vi "Main On Compile Action VI_Parse BC.vi"(7 "Autocreate Rx timestamp chans?":bool, 8 "error in":errorcluster, 10 "Channel Ref":u64, 11 "Device Item Ref in":T2 format="%.0x") -> (0 "error out":errorcluster, 2 "Channel Ref":u64, 3 "BC":T1 {"Acyclic Frames Trigger Channels Refs" format="%.0x"; "Command Channels Refs" format="%.0x"; "messages"."Timestamp Channel Data Reference" format="%.0x"; "messages"."Status Channel Data Refs" format="%.0x"; "messages"."Words Item Refs" format="%.0x"; "messages"."Words Block Data Refs"."Data Reference" format="%.0x"})   [LabVIEW 2017, in "Ballard 1553 System Explorer.lvlib"]
uses:
  Ballard 1553 System Explorer.lvlib
  <vilib>/NI Veristand/Custom Device API/Custom Device Item Ref.ctl
  Shared/Controls and Global/RT BC.ctl
  Shared/Controls and Global/RT Message.ctl
  Shared/Controls and Global/RT messageType.ctl
  Shared/Controls and Global/RT CWD1.ctl
  Shared/Controls and Global/RT CWD2.ctl
  <vilib>/NI Veristand/Custom Device API/Data Reference.ctl
  <vilib>/NI Veristand/Custom Device API/Block Data Reference.ctl
  Parse XML Ballard/Ballard_messageType.ctl
  Parse XML Ballard/Ballard_CWD1.ctl
  Parse XML Ballard/Ballard_CWD2.ctl
  <vilib>/NI Veristand/Custom Device API/Data Access Type.ctl
  Shared/Controls and Global/Global.vi
  <vilib>/NI Veristand/Custom Device Tools/Custom Device Utility Library/NI VeriStand - Search for Item by GUID.vi
  <vilib>/NI Veristand/Custom Device API/Get Item Property (I32).vi
  <vilib>/NI Veristand/Custom Device API/Get Item Property (String).vi
  <vilib>/NI Veristand/Custom Device Tools/Custom Device Utility Library/NI VeriStand - Search for Item by Name.vi
  <vilib>/NI Veristand/Custom Device Tools/Custom Device Utility Library/NI VeriStand - Search for All Items by GUID.vi
  <vilib>/NI Veristand/Custom Device API/Get Item Property (U16).vi
  <vilib>/NI Veristand/Custom Device API/Get Item Property (Variant).vi
  Shared/Ballard 1553 Shared.lvlib
  <vilib>/NI VeriStand/Custom Device Tools/Custom Device Utility Library/Custom Device Utility Library.lvlib
  <vilib>/NI VeriStand/Custom Device API/Custom Device API.lvlib
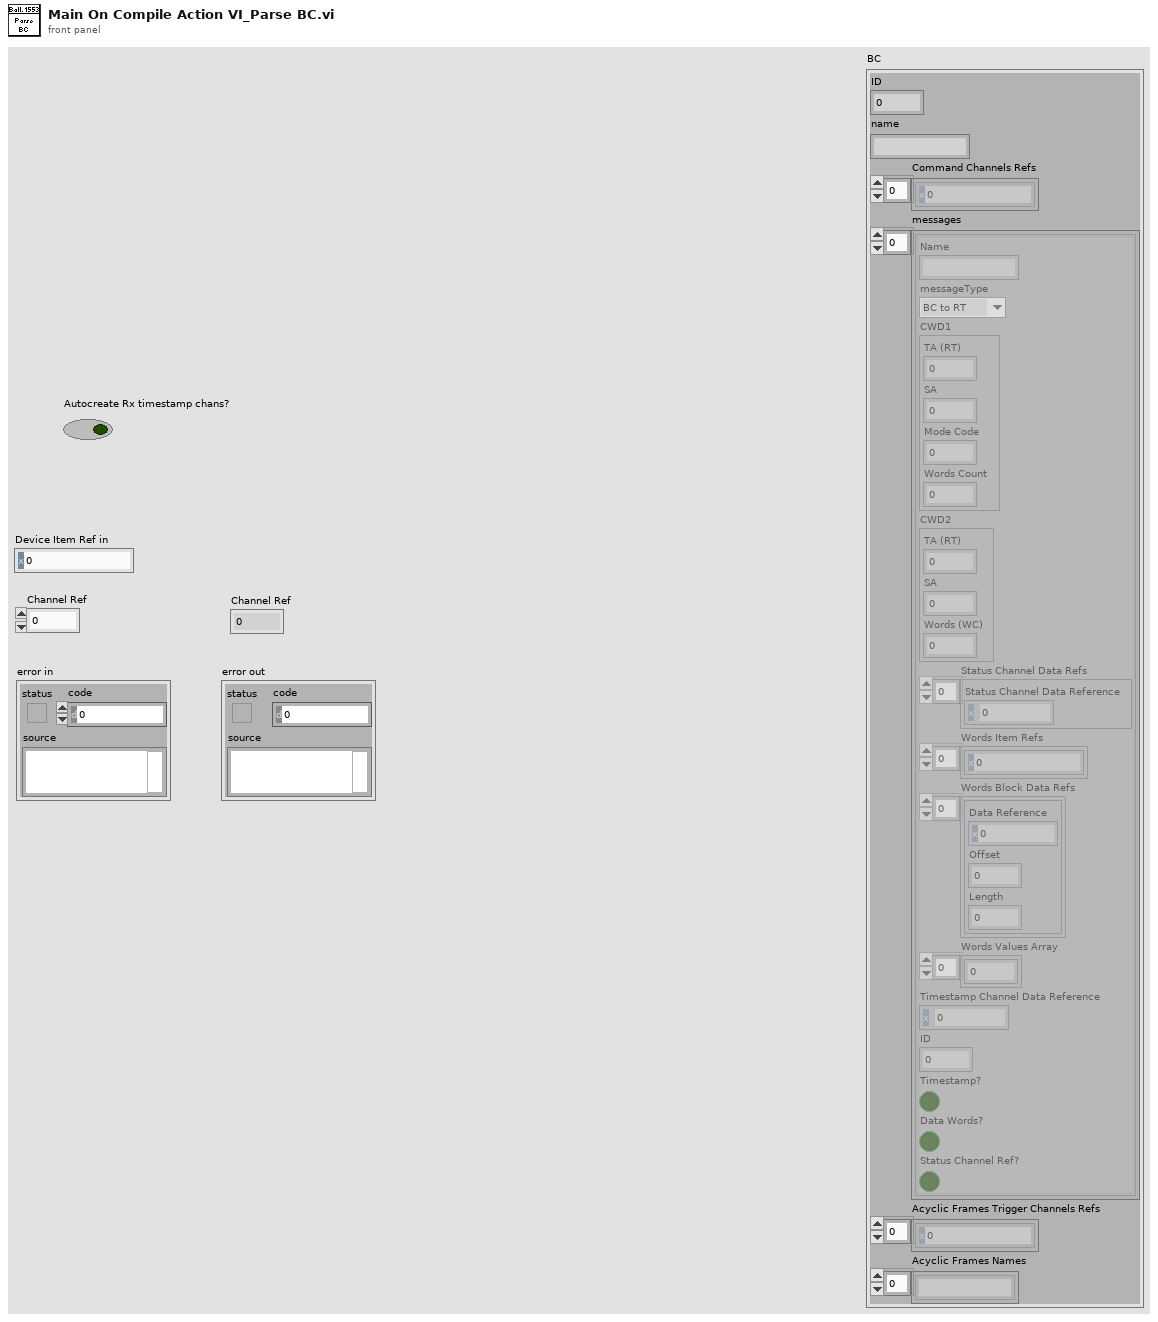
[diagram p1: front panel]
types:
  T1 = typedef "Ballard 1553 Shared.lvlib/RT BC.ctl" = cluster{"ID":i32, "name":string, "Command Channels Refs":T2[], "messages":T3[], "Acyclic Frames Trigger Channels Refs":T2[], "Acyclic Frames Names":string[]}
  T2 = typedef "Custom Device API.lvlib/Custom Device Item Ref.ctl" = u64
  T3 = typedef "Ballard 1553 Shared.lvlib/RT Message.ctl" = cluster{"Name":string, "messageType":T4, "CWD1":T5, "CWD2":T6, "Status Channel Data Refs":T7[], "Words Item Refs":T2[], "Words Block Data Refs":T8[], "Words Values Array":u16[], "Timestamp Channel Data Reference":T7, "ID":i32, "Timestamp?":bool, "Data Words?":bool, "Status Channel Ref?":bool}
  T4 = typedef "Ballard 1553 Shared.lvlib/RT messageType.ctl" = enum16{"BC to RT", "RT to BC", "RT to RT", "MC (Rx)", "MC (Tx)"}
  T5 = typedef "Ballard 1553 Shared.lvlib/RT CWD1.ctl" = cluster{"TA (RT)":i8, "SA":i8, "Mode Code":i8, "Words Count":i8}
  T6 = typedef "Ballard 1553 Shared.lvlib/RT CWD2.ctl" = cluster{"TA (RT)":i8, "SA":i8, "Words (WC)":i8}
  T7 = typedef "Custom Device API.lvlib/Data Reference.ctl" = i32
  T8 = typedef "Custom Device API.lvlib/Block Data Reference.ctl" = cluster{"Data Reference":T7, "Offset":u64, "Length":u64}
  T9 = typedef "Ballard 1553 System Explorer.lvlib/Ballard_CWD2.ctl" = cluster{"TA (RT)":i8, "SA":i8, "Words (WC)":i8}
  T10 = typedef "Ballard 1553 System Explorer.lvlib/Ballard_CWD1.ctl" = cluster{"TA (RT)":i8, "SA":i8, "Mode Code":i8, "Words Count":i8}
  T11 = typedef "Ballard 1553 System Explorer.lvlib/Ballard_messageType.ctl" = enum16{"BC to RT", "RT to BC", "RT to RT", "MC (Rx)", "MC (Tx)"}
  T12 = typedef "Custom Device API.lvlib/Data Access Type.ctl" = enum16{"Read", "Write"}
  T13 = typedef "Custom Device API.lvlib/Custom Device Item Info.ctl" = cluster{"Name":string, "Is Channel":bool, "GUID":string, "Is Waveform":bool}
  T14 = typedef "Custom Device API.lvlib/Custom Device Channel.ctl" = cluster{"Type":T15, "Units":string, "Default Value":dbl, "Faultable":bool, "Scalable":bool}
  T15 = typedef "Custom Device API.lvlib/Custom Device Channel Type.ctl" = enum16{"Input", "Output"}
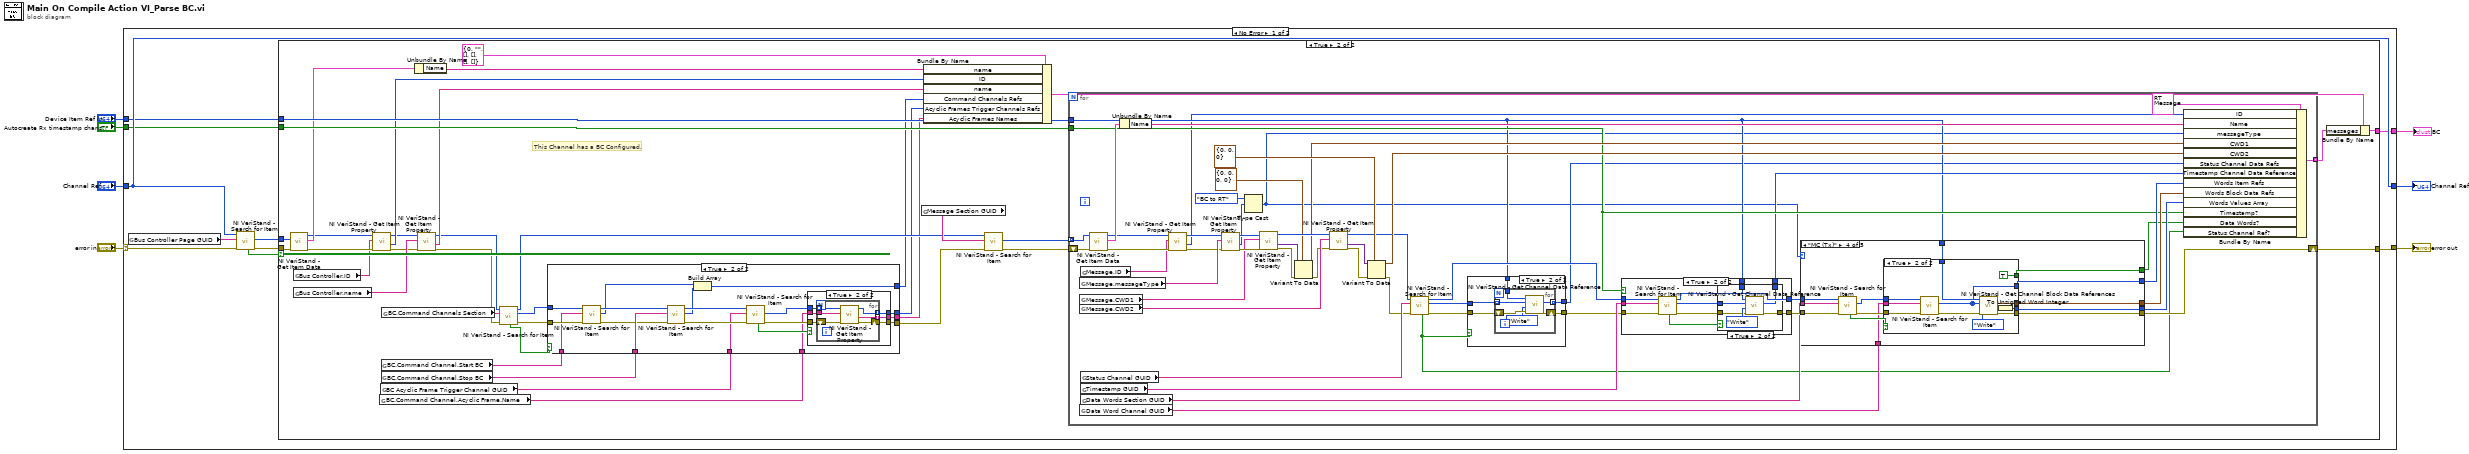
[diagram p0: block diagram]
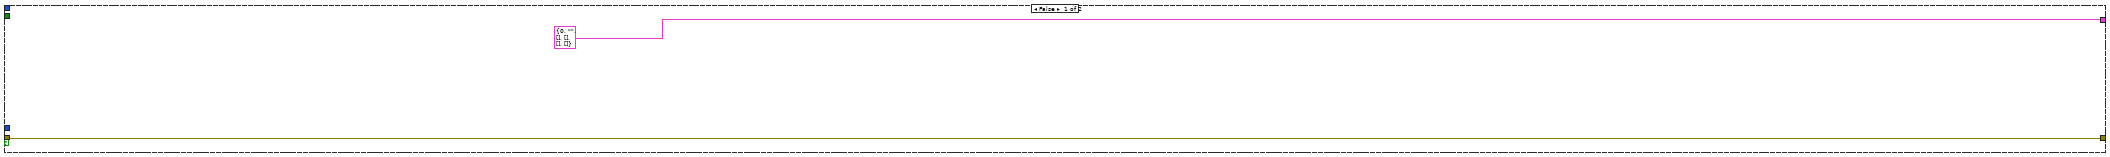
[diagram p2: hidden frame]
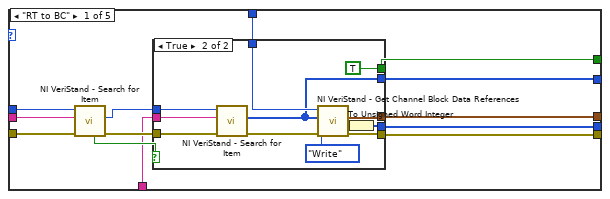
[diagram p6: hidden frame]
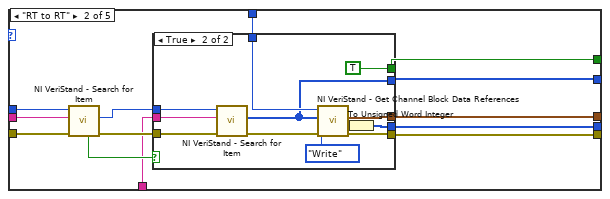
[diagram p8: hidden frame]
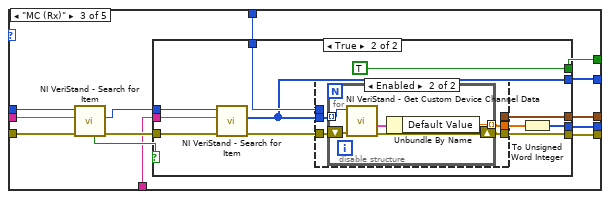
[diagram p10: hidden frame]
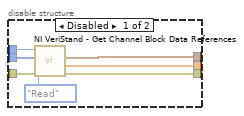
[diagram p12: hidden frame]
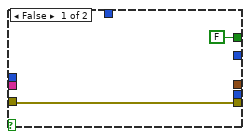
[diagram p13: hidden frame]
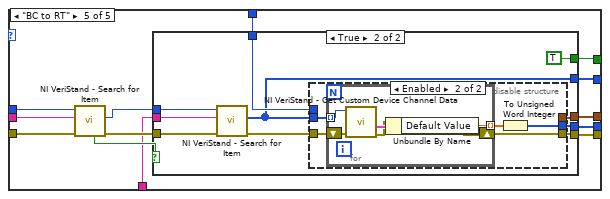
[diagram p14: hidden frame]
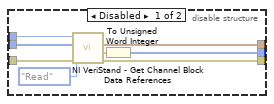
[diagram p16: hidden frame]
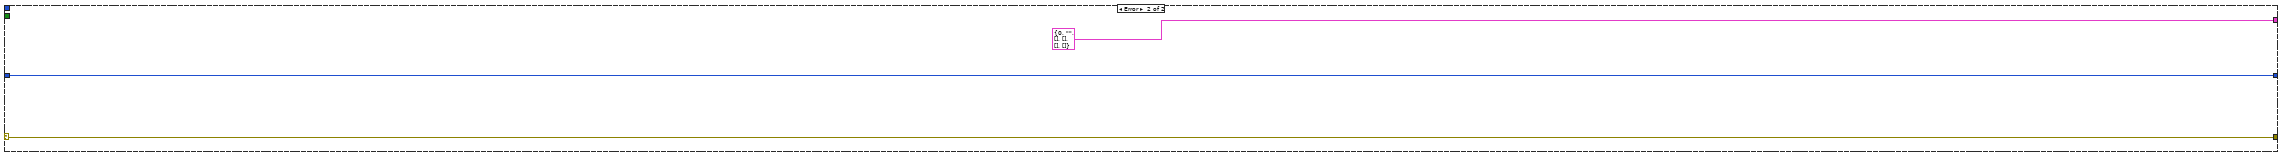
[diagram p19: hidden frame]
diagram:
  n1 = case shown="No Error" "error in" {
    selector: "error in" -> [w16 w338]
    tunnel: [w17 w338] -> w6
    tunnel: "Channel Ref" -> [w14 w337]
    tunnel: [w14 w337] -> w4
    tunnel: "Autocreate Rx timestamp chans?" -> [w10 _]
    tunnel: "Device Item Ref in" -> [w9 _]
    tunnel: [w8 T1 {"ID"=0, "name"="", "Command Channels Refs"=[], "messages"=[], "Acyclic Frames Trigger Channels Refs"=[], "Acyclic Frames Names"=[]} ("BC")] -> w1
    frame No Error {
      n2 = global read "Global.vi" "Bus Controller Page GUID"() -> (w15:string)
      n3 = call-poly <vilib>:"NI VeriStand - Search for Item.vi"("error in"=w16, "Item GUID"=w15, "Section Ref in"=w14) -> ("error out"=w13:errorcluster, "Item Ref"=w11:T2, "Found"=w12:bool)  [unwired: 5 in, 1 out]
      n4 = case shown="True" w12 {
        tunnel: w13 -> [w19 w39]
        tunnel: w11 -> [_ w40]
        tunnel: w10 -> [_ w53]
        tunnel: [w19 w52] -> w17
        tunnel: w9 -> [_ w51]
        tunnel: [T1 {"ID"=0, "name"="", "Command Channels Refs"=[], "messages"=[], "Acyclic Frames Trigger Channels Refs"=[], "Acyclic Frames Names"=[]} ("BC") w49] -> w8
        frame False {
        }
        frame True {
          # "This Channel has a BC Configured."
          n5 = call <vilib>:"NI VeriStand - Get Item Data.vi"("error in (no error)"=w39, "Item Ref in"=w40) -> ("error out"=w33:errorcluster, "Item Info"=w38:T13, "Item Ref out"=w34:T2)  [unwired: 6 in, 1 out]
          n6 = global read "Global.vi" "Bus Controller.ID"() -> (w32:string)
          n7 = global read "Global.vi" "Bus Controller.name"() -> (w29:string)
          n8 = call-poly <vilib>:"NI VeriStand - Get Item Property.vi"("error in (no error)"=w33, "Property Name"=w32, "Item Ref in"=w34) -> ("error out"=w28:errorcluster, "Value"=w31:i32, "Item Ref out"=w30:T2)  [unwired: 5 in, 1 out]
          n9 = global read "Global.vi" "BC.Command Channel.Acyclic Frame.Name"() -> (w22:string)
          n10 = global read "Global.vi" "BC Acyclic Frame Trigger Channel GUID"() -> (w23:string)
          n11 = global read "Global.vi" "BC.Command Channel.Start BC"() -> (w43:string)
          n12 = global read "Global.vi" "BC.Command Channel.Stop BC"() -> (w42:string)
          n13 = global read "Global.vi" "BC.Command Channels Section"() -> (w45:string)
          n14 = Unbundle By Name(w38) -> ("Name"=w36:string)
          n15 = call-poly <vilib>:"NI VeriStand - Get Item Property.vi"("error in (no error)"=w28, "Property Name"=w29, "Item Ref in"=w30) -> ("error out"=w27:errorcluster, "Value"=w26:string, "Item Ref out"=w24:T2)  [unwired: 5 in, 1 out]
          n16 = call-poly <vilib>:"NI VeriStand - Search for Item.vi"("error in"=w27, "Item Name"=w45, "Section Ref in"=w24) -> ("error out"=w46:errorcluster, "Item Ref"=w48:T2, "Section Ref out"=w41:T2, "Found"=w47:bool)  [unwired: 5 in]
          n17 = case shown="True" w47 {
            tunnel: w46 -> [w57 w76]
            tunnel: w48 -> [_ w75]
            tunnel: w43 -> [_ w74]
            tunnel: w42 -> [_ w73]
            tunnel: [w57 w61] -> w44
            tunnel: [_ w70] -> w25
            tunnel: [_ w60] -> w21
            tunnel: w23 -> [_ w68]
            tunnel: [_ w59] -> w20
            tunnel: w22 -> [_ w58]
            frame False {
            }
            frame True {
              n18 = call-poly <vilib>:"NI VeriStand - Search for Item.vi"("error in"=w76, "Item Name"=w74, "Section Ref in"=w75) -> ("error out"=w71:errorcluster, "Item Ref"=w66:T2, "Section Ref out"=w72:T2)  [unwired: 5 in, 1 out]
              n19 = call-poly <vilib>:"NI VeriStand - Search for Item.vi"("error in"=w71, "Item Name"=w73, "Section Ref in"=w72) -> ("error out"=w69:errorcluster, "Item Ref"=w65:T2, "Section Ref out"=w67:T2)  [unwired: 5 in, 1 out]
              n20 = Build Array(w66, w65) -> (w70:T2[])
              n21 = call-poly <vilib>:"NI VeriStand - Search for Item.vi"("error in"=w69, "Item GUID"=w68, "Section Ref in"=w67) -> ("error out"=w63:errorcluster, "Item Refs"=w62:T2[], "Found"=w64:bool)  [unwired: 5 in, 1 out]
              n22 = case shown="True" w64 {
                tunnel: w63 -> [w78 w83]
                tunnel: w62 -> [w77 w84]
                tunnel: [w78 w82] -> w61
                tunnel: [w77 w81] -> w60
                tunnel: [_ w80] -> w59
                tunnel: w58 -> [_ w79]
                frame False {
                }
                frame True {
                  n23 = for {
                    tunnel: w84 -> [w90] mode=indexing
                    shift-right: [w88] -> w82
                    shift-left: w83 -> [w89]
                    tunnel: [w87] -> w81 mode=indexing
                    tunnel: [w86] -> w80 mode=indexing
                    tunnel: w79 -> [w85]
                    n24 = call-poly <vilib>:"NI VeriStand - Get Item Property.vi"("error in (no error)"=w89, "Property Name"=w85, "Item Ref in"=w90) -> ("error out"=w88:errorcluster, "Value"=w86:string, "Item Ref out"=w87:T2)  [unwired: 5 in, 1 out]
                  }
                }
              }
            }
          }
          n25 = global read "Global.vi" "Message Section GUID"() -> (w56:string)
          n26 = Bundle By Name(cluster=T1 {"ID"=0, "name"="", "Command Channels Refs"=[], "messages"=[], "Acyclic Frames Trigger Channels Refs"=[], "Acyclic Frames Names"=[]} ("BC"), "name"=w36, "ID"=w31, "name"=w26, "Command Channels Refs"=w25, "Acyclic Frames Trigger Channels Refs"=w21, "Acyclic Frames Names"=w20) -> (w35:T1)
          n27 = call-poly <vilib>:"NI VeriStand - Search for Item.vi"("error in"=w44, "Item GUID"=w56, "Section Ref in"=w41) -> ("error out"=w55:errorcluster, "Item Refs"=w54:T2[])  [unwired: 5 in, 2 out]
          n28 = for {
            tunnel: w54 -> [w119] mode=indexing
            shift-right: [w121] -> w52
            shift-left: w55 -> [w120]
            tunnel: w53 -> [w102]
            tunnel: w51 -> [w94]
            tunnel: [w111] -> w50 mode=indexing
            n29 = global read "Global.vi" "Message.messageType"() -> (w139:string)
            n30 = global read "Global.vi" "Message.CWD1"() -> (w138:string)
            n31 = global read "Global.vi" "Message.CWD2"() -> (w137:string)
            n32 = global read "Global.vi" "Data Word Channel GUID"() -> (w122:string)
            n33 = global read "Global.vi" "Message.ID"() -> (w105:string)
            n34 = global read "Global.vi" "Status Channel GUID"() -> (w127:string)
            n35 = global read "Global.vi" "Timestamp GUID"() -> (w126:string)
            n36 = global read "Global.vi" "Data Words Section GUID"() -> (w123:string)
            n37 = call <vilib>:"NI VeriStand - Get Item Data.vi"("error in (no error)"=w120, "Item Ref in"=w119) -> ("error out"=w106:errorcluster, "Item Info"=w118:T13, "Item Ref out"=w107:T2)  [unwired: 6 in, 1 out]
            n38 = Unbundle By Name(w118) -> ("Name"=w117:string)
            n39 = call-poly <vilib>:"NI VeriStand - Get Item Property.vi"("error in (no error)"=w106, "Property Name"=w105, "Item Ref in"=w107) -> ("error out"=w104:errorcluster, "Value"=w91:i32, "Item Ref out"=w103:T2)  [unwired: 5 in, 1 out]
            n40 = call-poly <vilib>:"NI VeriStand - Get Item Property.vi"("error in (no error)"=w104, "Property Name"=w139, "Item Ref in"=w103) -> ("error out"=w142:errorcluster, "Value"=w131:u16, "Item Ref out"=w140:T2)  [unwired: 5 in, 1 out]
            n41 = Type Cast(type=Ballard_messageType."BC to RT" ("messageType"), x=w131) -> (*(type *) &x=w92:T11)
            n42 = call-poly <vilib>:"NI VeriStand - Get Item Property.vi"("error in (no error)"=w142, "Property Name"=w138, "Item Ref in"=w140) -> ("error out"=w136:errorcluster, "Value"=w133:variant, "Item Ref out"=w141:T2)  [unwired: 5 in, 1 out]
            n43 = Variant To Data(error in=w136, type=T10 {"TA (RT)"=0, "SA"=0, "Mode Code"=0, "Words Count"=0} ("CWD1"), Variant=w133) -> (data=w116:T10, error out=w134:errorcluster)
            n44 = call-poly <vilib>:"NI VeriStand - Get Item Property.vi"("error in (no error)"=w134, "Property Name"=w137, "Item Ref in"=w141) -> ("error out"=w135:errorcluster, "Value"=w132:variant, "Item Ref out"=w110:T2)  [unwired: 5 in, 1 out]
            n45 = Variant To Data(error in=w135, type=T9 {"TA (RT)"=0, "SA"=0, "Words (WC)"=0} ("CWD1"), Variant=w132) -> (data=w115:T9, error out=w109:errorcluster)
            n46 = call-poly <vilib>:"NI VeriStand - Search for Item.vi"("error in"=w109, "Item GUID"=w127, "Section Ref in"=w110) -> ("error out"=w98:errorcluster, "Item Refs"=w96:T2[], "Section Ref out"=w95:T2, "Found"=w99:bool)  [unwired: 5 in]
            n47 = case shown="True" w99 {
              tunnel: w98 -> [w143 w148]
              tunnel: [w143 w147] -> w97
              tunnel: w96 -> [_ w145]
              tunnel: w94 -> [_ w146]
              tunnel: [_ w144] -> w93
              frame False {
              }
              frame True {
                n48 = for {
                  tunnel: w146 -> [w152]
                  shift-right: [w153] -> w147
                  shift-left: w148 -> [w154]
                  tunnel: w145 -> [w150] mode=indexing
                  tunnel: [w149] -> w144 mode=indexing
                  n49 = call <vilib>:"NI VeriStand - Get Channel Data Reference.vi"("error in (no error)"=w154, "Access"=Data_Access_Type."Write", "Channel Ref in"=w150, "Device Ref in"=w152) -> ("error out"=w153:errorcluster, "Channel Data Reference"=w149:T7)  [unwired: 5 in, 1 out]
                }
              }
            }
            n50 = case shown="True" w102 {
              tunnel: w95 -> [w317 w328]
              tunnel: w97 -> [w318 w327]
              tunnel: [w318 w325] -> w125
              tunnel: w126 -> [_ w326]
              tunnel: [w317 w323] -> w124
              tunnel: w94 -> [_ w322]
              tunnel: [_ w320] -> w100
              frame False {
              }
              frame True {
                n51 = call-poly <vilib>:"NI VeriStand - Search for Item.vi"("error in"=w327, "Item GUID"=w326, "Section Ref in"=w328) -> ("error out"=w324:errorcluster, "Item Ref"=w321:T2, "Section Ref out"=w323:T2, "Found"=w319:bool)  [unwired: 5 in]
                n52 = case shown="True" w319 {
                  tunnel: [w329 w334] -> w325
                  tunnel: w324 -> [w329 w333]
                  tunnel: w322 -> [_ w332]
                  tunnel: w321 -> [_ w331]
                  tunnel: [_ w330] -> w320
                  frame False {
                  }
                  frame True {
                    n53 = call <vilib>:"NI VeriStand - Get Channel Data Reference.vi"("error in (no error)"=w333, "Access"=Data_Access_Type."Write", "Channel Ref in"=w331, "Device Ref in"=w332) -> ("error out"=w334:errorcluster, "Channel Data Reference"=w330:T7)  [unwired: 5 in, 1 out]
                  }
                }
              }
            }
            n54 = case shown="\"MC (Tx)\"" w92 {
              tunnel: w125 -> [w167 w193 w219 w260 w287]
              tunnel: w124 -> [w166 w192 w218 w259 w286]
              tunnel: w123 -> [w165 w191 w217 w258 w285]
              tunnel: w122 -> [w161 w187 w213 w254 w281]
              tunnel: [w160 w186 w212 w253 w280] -> w121
              tunnel: w94 -> [w159 w185 w211 w252 w279]
              tunnel: [w158 w184 w210 w251 w278] -> w113
              tunnel: [w157 w183 w209 w250 w277] -> w112
              tunnel: [w156 w182 w208 w249 w276] -> w114
              tunnel: [w155 w181 w207 w248 w275] -> w101
              frame "RT to BC" {
                n55 = call-poly <vilib>:"NI VeriStand - Search for Item.vi"("error in"=w167, "Item GUID"=w165, "Section Ref in"=w166) -> ("error out"=w164:errorcluster, "Item Ref"=w162:T2, "Found"=w163:bool)  [unwired: 5 in, 1 out]
                n56 = case shown="True" w163 {
                  tunnel: w164 -> [w168 w178]
                  tunnel: w162 -> [_ w180]
                  tunnel: w161 -> [_ w179]
                  tunnel: [w168 w176] -> w160
                  tunnel: w159 -> [_ w175]
                  tunnel: [_ w173] -> w156
                  tunnel: [_ w172] -> w158
                  tunnel: [_ w170] -> w157
                  tunnel: [_ TRUE] -> w155
                  frame False {
                  }
                  frame True {
                    n57 = call-poly <vilib>:"NI VeriStand - Search for Item.vi"("error in"=w178, "Item GUID"=w179, "Section Ref in"=w180) -> ("error out"=w177:errorcluster, "Item Refs"=w173:T2[])  [unwired: 5 in, 2 out]
                    n58 = call <vilib>:"NI VeriStand - Get Channel Block Data References.vi"("error in (no error)"=w177, "Access"=Data_Access_Type."Write", "Channel Refs"=w173, "Device Ref in"=w175) -> ("error out"=w176:errorcluster, "Values Array"=w171:dbl[], "Block Data Refs"=w172:T8[])  [unwired: 4 in, 1 out]
                    n59 = To Unsigned Word Integer(number=w171) -> (unsigned 16bit integer=w170:u16[])
                  }
                }
              }
              frame "RT to RT" {
                n60 = call-poly <vilib>:"NI VeriStand - Search for Item.vi"("error in"=w193, "Item GUID"=w191, "Section Ref in"=w192) -> ("error out"=w190:errorcluster, "Item Ref"=w188:T2, "Found"=w189:bool)  [unwired: 5 in, 1 out]
                n61 = case shown="True" w189 {
                  tunnel: w190 -> [w194 w204]
                  tunnel: w188 -> [_ w206]
                  tunnel: w187 -> [_ w205]
                  tunnel: [w194 w202] -> w186
                  tunnel: w185 -> [_ w201]
                  tunnel: [_ w195] -> w182
                  tunnel: [_ w199] -> w184
                  tunnel: [_ w197] -> w183
                  tunnel: [_ TRUE] -> w181
                  frame False {
                  }
                  frame True {
                    n62 = call-poly <vilib>:"NI VeriStand - Search for Item.vi"("error in"=w204, "Item GUID"=w205, "Section Ref in"=w206) -> ("error out"=w203:errorcluster, "Item Refs"=w195:T2[])  [unwired: 5 in, 2 out]
                    n63 = call <vilib>:"NI VeriStand - Get Channel Block Data References.vi"("error in (no error)"=w203, "Access"=Data_Access_Type."Write", "Channel Refs"=w195, "Device Ref in"=w201) -> ("error out"=w202:errorcluster, "Values Array"=w198:dbl[], "Block Data Refs"=w199:T8[])  [unwired: 4 in, 1 out]
                    n64 = To Unsigned Word Integer(number=w198) -> (unsigned 16bit integer=w197:u16[])
                  }
                }
              }
              frame "MC (Rx)" {
                n65 = call-poly <vilib>:"NI VeriStand - Search for Item.vi"("error in"=w219, "Item GUID"=w217, "Section Ref in"=w218) -> ("error out"=w216:errorcluster, "Item Ref"=w214:T2, "Found"=w215:bool)  [unwired: 5 in, 1 out]
                n66 = case shown="True" w215 {
                  tunnel: w216 -> [w220 w229]
                  tunnel: w214 -> [_ w231]
                  tunnel: w213 -> [_ w230]
                  tunnel: [w220 w227] -> w212
                  tunnel: w211 -> [_ w226]
                  tunnel: [_ w225] -> w208
                  tunnel: [_ w224] -> w210
                  tunnel: [_ w222] -> w209
                  tunnel: [_ TRUE] -> w207
                  frame False {
                  }
                  frame True {
                    n67 = call-poly <vilib>:"NI VeriStand - Search for Item.vi"("error in"=w229, "Item GUID"=w230, "Section Ref in"=w231) -> ("error out"=w228:errorcluster, "Item Refs"=w225:T2[])  [unwired: 5 in, 2 out]
                    n68 = disable-structure shown="Enabled" {
                      disable-tunnel: w228 -> [w238 w241]
                      disable-tunnel: [w237 w240] -> w227
                      disable-tunnel: w226 -> [w236 _]
                      disable-tunnel: w225 -> [w234 w242]
                      disable-tunnel: [w233 _] -> w224
                      disable-tunnel: [w232 w239] -> w223
                      frame Disabled {
                        n69 = call <vilib>:"NI VeriStand - Get Channel Block Data References.vi"("error in (no error)"=w238, "Access"=Data_Access_Type."Read", "Channel Refs"=w234, "Device Ref in"=w236) -> ("error out"=w237:errorcluster, "Values Array"=w232:dbl[], "Block Data Refs"=w233:T8[])  [unwired: 4 in, 1 out]
                      }
                      frame Enabled {
                        n70 = for {
                          tunnel: [w243] -> w239 mode=indexing
                          shift-right: [w244] -> w240
                          shift-left: w241 -> [w247]
                          tunnel: w242 -> [w245] mode=indexing
                          n71 = call <vilib>:"NI VeriStand - Get Custom Device Channel Data.vi"("error in (no error)"=w247, "Channel Ref in"=w245) -> ("error out"=w244:errorcluster, "Channel"=w246:T14)  [unwired: 4 in, 4 out]
                          n72 = Unbundle By Name(w246) -> ("Default Value"=w243:dbl)
                        }
                      }
                    }
                    n73 = To Unsigned Word Integer(number=w223) -> (unsigned 16bit integer=w222:u16[])
                  }
                }
              }
              frame "MC (Tx)" {
                n74 = call-poly <vilib>:"NI VeriStand - Search for Item.vi"("error in"=w260, "Item GUID"=w258, "Section Ref in"=w259) -> ("error out"=w257:errorcluster, "Item Ref"=w255:T2, "Found"=w256:bool)  [unwired: 5 in, 1 out]
                n75 = case shown="True" w256 {
                  tunnel: w257 -> [w262 w272]
                  tunnel: w255 -> [_ w274]
                  tunnel: w254 -> [_ w273]
                  tunnel: [w262 w270] -> w253
                  tunnel: w252 -> [_ w269]
                  tunnel: [_ w267] -> w249
                  tunnel: [_ w266] -> w251
                  tunnel: [_ w264] -> w250
                  tunnel: [FALSE TRUE] -> w248
                  frame False {
                  }
                  frame True {
                    n76 = call-poly <vilib>:"NI VeriStand - Search for Item.vi"("error in"=w272, "Item GUID"=w273, "Section Ref in"=w274) -> ("error out"=w271:errorcluster, "Item Refs"=w267:T2[])  [unwired: 5 in, 2 out]
                    n77 = call <vilib>:"NI VeriStand - Get Channel Block Data References.vi"("error in (no error)"=w271, "Access"=Data_Access_Type."Write", "Channel Refs"=w267, "Device Ref in"=w269) -> ("error out"=w270:errorcluster, "Values Array"=w265:dbl[], "Block Data Refs"=w266:T8[])  [unwired: 4 in, 1 out]
                    n78 = To Unsigned Word Integer(number=w265) -> (unsigned 16bit integer=w264:u16[])
                  }
                }
              }
              frame "BC to RT" {
                n79 = call-poly <vilib>:"NI VeriStand - Search for Item.vi"("error in"=w287, "Item GUID"=w285, "Section Ref in"=w286) -> ("error out"=w284:errorcluster, "Item Ref"=w282:T2, "Found"=w283:bool)  [unwired: 5 in, 1 out]
                n80 = case shown="True" w283 {
                  tunnel: w284 -> [w288 w296]
                  tunnel: w282 -> [_ w298]
                  tunnel: w281 -> [_ w297]
                  tunnel: [w288 w294] -> w280
                  tunnel: w279 -> [_ w293]
                  tunnel: [_ w292] -> w276
                  tunnel: [_ w291] -> w278
                  tunnel: [_ w290] -> w277
                  tunnel: [_ TRUE] -> w275
                  frame False {
                  }
                  frame True {
                    n81 = call-poly <vilib>:"NI VeriStand - Search for Item.vi"("error in"=w296, "Item GUID"=w297, "Section Ref in"=w298) -> ("error out"=w295:errorcluster, "Item Refs"=w292:T2[])  [unwired: 5 in, 2 out]
                    n82 = disable-structure shown="Enabled" {
                      disable-tunnel: w295 -> [w306 w311]
                      disable-tunnel: [w305 w310] -> w294
                      disable-tunnel: w293 -> [w304 _]
                      disable-tunnel: w292 -> [w302 w307]
                      disable-tunnel: [w301 _] -> w291
                      disable-tunnel: [w299 w308] -> w290
                      frame Disabled {
                        n83 = call <vilib>:"NI VeriStand - Get Channel Block Data References.vi"("error in (no error)"=w306, "Access"=Data_Access_Type."Read", "Channel Refs"=w302, "Device Ref in"=w304) -> ("error out"=w305:errorcluster, "Values Array"=w300:dbl[], "Block Data Refs"=w301:T8[])  [unwired: 4 in, 1 out]
                        n84 = To Unsigned Word Integer(number=w300) -> (unsigned 16bit integer=w299:u16[])
                      }
                      frame Enabled {
                        n85 = for {
                          tunnel: [w312] -> w309 mode=indexing
                          shift-right: [w313] -> w310
                          shift-left: w311 -> [w316]
                          tunnel: w307 -> [w314] mode=indexing
                          n86 = call <vilib>:"NI VeriStand - Get Custom Device Channel Data.vi"("error in (no error)"=w316, "Channel Ref in"=w314) -> ("error out"=w313:errorcluster, "Channel"=w315:T14)  [unwired: 4 in, 4 out]
                          n87 = Unbundle By Name(w315) -> ("Default Value"=w312:dbl)
                        }
                        n88 = To Unsigned Word Integer(number=w309) -> (unsigned 16bit integer=w308:u16[])
                      }
                    }
                  }
                }
              }
            }
            n89 = Bundle By Name(cluster=T3 {"Name"="", "messageType"=enum."BC to RT", "CWD1"={"TA (RT)"=0, "SA"=0, "Mode Code"=0, "Words Count"=0}, "CWD2"={"TA (RT)"=0, "SA"=0, "Words (WC)"=0}, "Status Channel Data Refs"=[], "Words Item Refs"=[], "Words Block Data Refs"=[], "Words Values Array"=[], "Timestamp Channel Data Reference"=0, "ID"=0, "Timestamp?"=FALSE, "Data Words?"=FALSE, "Status Channel Ref?"=FALSE} ("output cluster"), "ID"=w91, "Name"=w117, "messageType"=w92, "CWD1"=w116, "CWD2"=w115, "Status Channel Data Refs"=w93, "Timestamp Channel Data Reference"=w100, "Words Item Refs"=w114, "Words Block Data Refs"=w113, "Words Values Array"=w112, "Timestamp?"=w102, "Data Words?"=w101, "Status Channel Ref?"=w99) -> (w111:T3)
          }
          n90 = Bundle By Name(cluster=w35, "messages"=w50) -> (w49:T1)
        }
      }
    }
    frame Error {
    }
  }
  "error out" <- w6
  "Channel Ref" <- w4
  "BC" <- w1
